vi "Switch Shutdown (Poly).vi"   [LabVIEW 2016, in "Hall Effect Library.lvlib"]
uses:
  Hall Effect Library.lvlib
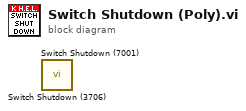
[diagram p0: block diagram]
diagram:
  n1 = call "Switch Shutdown (3706).vi"() -> ()  [unwired: 10 in, 2 out]
  n2 = call "Switch Shutdown (7001).vi"() -> ()  [unwired: 10 in, 2 out]
